vi "BMM LIN Set Para.vi"(6 "BreakSpace":i32, 7 "InterByteSpace":i32, 9 "BreakBits":u8, 10 "LINIndex":u8, 11 "DevHandle":i32) -> (3 "function return":i32)   [LabVIEW 2010, in "usb2bmm_lin.lvlib"]
doc: "int WINAPI BMM_LIN_SetPara(int DevHandle, unsigned char LINIndex, unsigned char BreakBits, int InterByteSpace, int BreakSpace);"
uses:
  usb2bmm_lin.lvlib
  USB2XXX/trunk/USB2XXX/USB2XXX/vs2019/Release/USB2XXX.dll
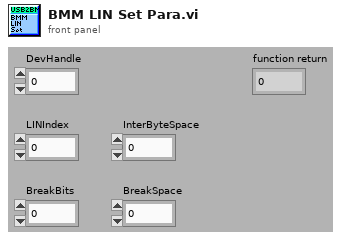
[diagram p1: front panel]
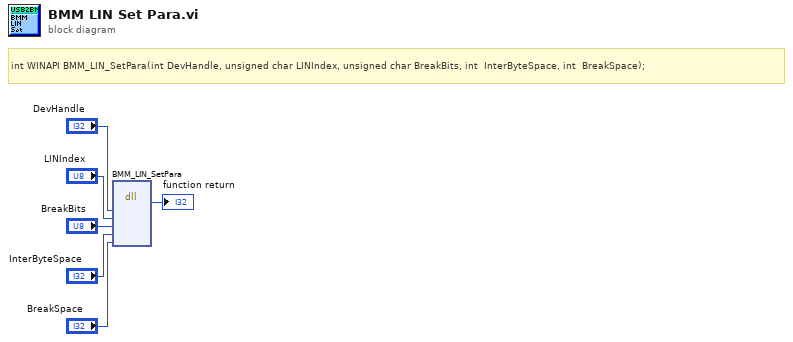
[diagram p0: block diagram]
diagram:
  # "int WINAPI BMM_LIN_SetPara(int DevHandle, unsigned char LINIndex, unsigned char BreakBits, int  InterByteSpace, int  BreakSpace);"
  n1 = dll-call lib="E:/Projects/USB2XXX/trunk/USB2XXX/USB2XXX/vs2019/Release/USB2XXX.*" fn="BMM_LIN_SetPara"("DevHandle"="DevHandle", "LINIndex"="LINIndex", "BreakBits"="BreakBits", "InterByteSpace"="InterByteSpace", "BreakSpace"="BreakSpace") -> (→"function return":i32)  [unwired: 8 in, 2 out]
